vi "transmisor serial.vi"() -> ()   [LabVIEW 2020]
uses:
  <vilib>/Instr/_visa.llb/VISA Configure Serial Port (Instr).vi
panel:
  in  "write buffer":string
  in  "Puerto Serial":refnum<visa-resource-name>
  in  "stop":bool
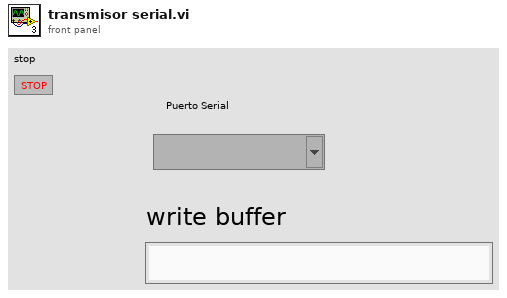
[diagram p1: front panel]
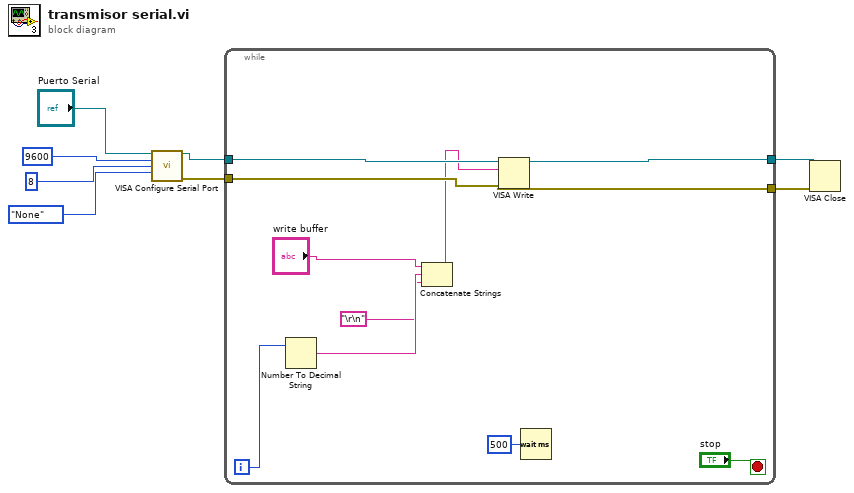
[diagram p0: block diagram]
diagram:
  n1 = call-poly "VISA Configure Serial Port"("VISA resource name"="Puerto Serial", "baud rate (9600)"=u32 9600, "data bits (8)"=u16 8, "parity (0:none)"=enum16{"None", "Odd", "Even", "Mark", "Space"}."None") -> ("VISA resource name out"=w4:refnum<visa-resource-name>, "error out"=w2:errorcluster)  [unwired: 10 in]
  n2 = while {
    tunnel: w4 -> [w17]
    tunnel: [w16] -> w3
    tunnel: w2 -> [w15]
    tunnel: [w14] -> w1
    i -> [w13]
    stop <- "stop" stop-if-true
    n3 = Number To Decimal String(number=w13) -> (decimal integer string=w11:string)  [unwired: 1 in]
    n4 = Concatenate Strings("write buffer", w11, "\r\n") -> (w9:string)
    n5 = VISA Write(VISA resource name=w17, write buffer=w9, error in (no error)=w15) -> (VISA resource name out=w16:refnum<visa-resource-name>, error out=w14:errorcluster)  [unwired: 1 out]
    n6 = Wait (ms)(milliseconds to wait=u32 500) -> ()  [unwired: 1 out]
  }
  n7 = VISA Close(VISA resource name=w3, error in (no error)=w1) -> ()  [unwired: 1 out]
